vi "ST example Test Joints.vi"() -> ()   [LabVIEW 2009]
panel:
  out "Angle":dbl[](array[numeric])
  out "Steps":i32[](array[numeric])
  out "At Location":bool
  out "STATUS\nREADY":bool
  out "Performed\nWAIST -1000":bool
  out "Proformed\nWAIST 1000":bool
  # "THIS IS A TEST ROUTINE FOR THE MOTIONS\nFIRST IT WILL INITIALIZE THE ROBOT AND THE CONTROLLER\nTHEN IT WILL EXERCISE A JOINT"
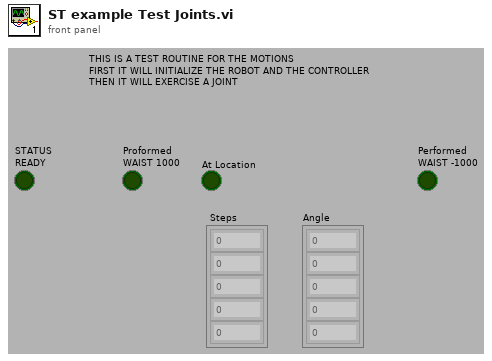
[diagram p1: front panel]
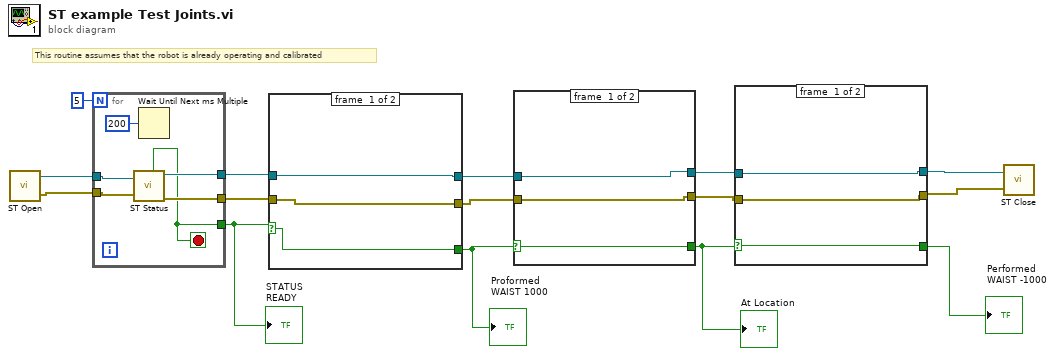
[diagram p0: block diagram]
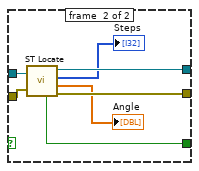
[diagram p2: hidden frame]
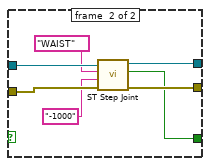
[diagram p3: hidden frame]
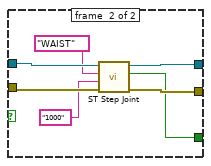
[diagram p4: hidden frame]
diagram:
  # "This routine assumes that the robot is already operating and calibrated"
  n1 = call "ST Open.vi"() -> ("VISA resource name out"=w14:refnum<visa-resource-name>, "error out"=w13:errorcluster)  [unwired: 1 in]
  n2 = for {
    N: 5 -> [_]
    tunnel: w14 -> [w20]
    tunnel: w13 -> [w21]
    tunnel: [w19] -> w11
    tunnel: [w18] -> w10
    tunnel: [w16] -> w12
    stop <- w16 stop-if-true
    n3 = call "ST Status.vi"("error in (no error)"=w21, "VISA resource name"=w20) -> ("error out"=w19:errorcluster, "VISA resource name out"=w18:refnum<visa-resource-name>, "Ready and OK"=w16:bool)  [unwired: 2 out]
    n4 = Wait Until Next ms Multiple(millisecond multiple=u32 200) -> ()  [unwired: 1 out]
  }
  "STATUS\nREADY" <- w12
  n5 = case shown="True" w12 {
    selector: w12 -> [w22 _]
    tunnel: w10 -> [w24 w31]
    tunnel: w11 -> [w23 w30]
    tunnel: [w24 w29] -> w1
    tunnel: [w23 w28] -> w2
    tunnel: [w22 w27] -> w3
    frame #0 {
    }
    frame #1 {
      n6 = call "ST Step Joint.vi"("error in (no error)"=w30, "STEPS"="1000", "Combo Box"="WAIST", "VISA resource name"=w31) -> ("error out"=w28:errorcluster, "Ready and OK"=w27:bool, "VISA resource name out"=w29:refnum<visa-resource-name>)  [unwired: 2 out]
    }
  }
  "Proformed\nWAIST 1000" <- w3
  n7 = case shown="True" w3 {
    selector: w3 -> [w32 _]
    tunnel: w1 -> [w34 w41]
    tunnel: w2 -> [w33 w40]
    tunnel: [w34 w39] -> w6
    tunnel: [w33 w38] -> w5
    tunnel: [w32 w37] -> w4
    frame #0 {
    }
    frame #1 {
      n8 = call "ST Locate.vi"("VISA resource name"=w41, "error in (no error)"=w40) -> ("Ready and OK"=w37:bool, "VISA resource name out"=w39:refnum<visa-resource-name>, "Steps"=→"Steps":i32[], "Angle"=→"Angle":dbl[], "error out"=w38:errorcluster)  [unwired: 1 out]
    }
  }
  "At Location" <- w4
  n9 = case shown="True" w4 {
    selector: w4 -> [w42 _]
    tunnel: w6 -> [w44 w51]
    tunnel: w5 -> [w43 w50]
    tunnel: [w44 w49] -> w8
    tunnel: [w43 w48] -> w7
    tunnel: [w42 w47] -> w9
    frame #0 {
    }
    frame #1 {
      n10 = call "ST Step Joint.vi"("error in (no error)"=w50, "STEPS"="-1000", "Combo Box"="WAIST", "VISA resource name"=w51) -> ("error out"=w48:errorcluster, "Ready and OK"=w47:bool, "VISA resource name out"=w49:refnum<visa-resource-name>)  [unwired: 2 out]
    }
  }
  "Performed\nWAIST -1000" <- w9
  n11 = call "ST Close.vi"("error in (no error)"=w7, "VISA resource name"=w8) -> ()
